vi "dscDIOOutputBit.vi"(6 "bit_val":enum8{"Lo", "Hi"}(ring), 8 "error in":errorcluster, 9 "bit":u8, 10 "port":u8, 11 "board":i16) -> (0 "error out":errorcluster, 3 "boardOut":i16)   [LabVIEW 2011, in "Diamond Universal Driver.lvlib"]
doc: "Sets the specified digital output bit of the specified port to the specified value (1 or 0) while leaving the other bits in their present states.\n\nSome boards (Diamond-MM, Diamond-MM-AT, Diamond-MM-16-AT, Opal-MM, Pearl-MM, Quartz-MM) do not have readback capability on the digital output ports. Therefore the driver maintains its own history of the last-written values to these ports, so that it can correctly modify only the bit of interest. In order for this function to work correctly, the driver must always know the present state of the digital output bits. This can only happen if you always use the driver for digital output operations. If you mix driver calls with direct I/O to the digital output ports, the bit operations can fail, since the driver will have no record of what your program has done directly."
uses:
  Diamond Universal Driver.lvlib
  Controls/error codes.ctl
  Instruments/WL OPC/Support/dlls/dscud.dll
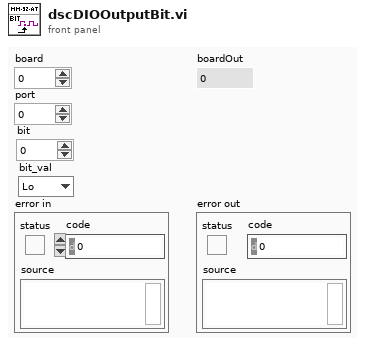
[diagram p1: front panel]
types:
  T1 = typedef "Diamond Universal Driver.lvlib/error codes.ctl" = enum8{"DE_NONE", "DE_HW_FAILURE", "DE_SW_FAILURE", "DE_HW_NOT_SUPPORTED", "DE_SW_NOT_SUPPORTED", "DE_INVALID_PARM", "DE_ALTERNATE_IN_PROGRESS", "DE_NONE_IN_PROGRESS", "DE_BUFFER_ROLLOVER", "DE_INVALID_ERROR_CODE", "DE_ALREADY_PAUSED", "DE_OVERFLOW", "DE_INVALID_FUNC", "DE_DSCUDH_INVALID", "DE_INVALID_BOARD", "DE_BOARD_LIMIT_REACHED", "DE_BOARD_BUSY", "DE_INVALID_WINDRVR_HANDLE", "DE_INVALID_WINDRVR_VERSION", "DE_BAD_WINDRVR_BOARD_INIT", "DE_OPERATION_TIMED_OUT", "DE_INVALID_WINDRVR_KP", "DE_THREAD_FAILURE"}
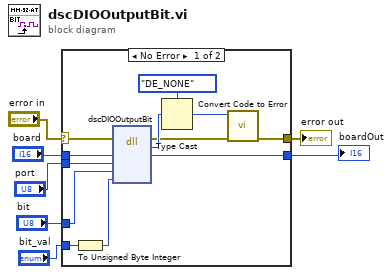
[diagram p0: block diagram]
diagram:
  n1 = case shown="No Error" "error in" {
    selector: "error in" -> [w16 w21]
    tunnel: "board" -> [w14 w20]
    tunnel: [w13 w20] -> w5
    tunnel: [w12 w21] -> w4
    tunnel: "port" -> [w11 _]
    tunnel: "bit" -> [w10 _]
    tunnel: "bit_val" -> [w9 _]
    frame No Error {
      n2 = To Unsigned Byte Integer(number=w9) -> (unsigned 8bit integer=w8:u8)
      n3 = dll-call lib="C:/Users/mrichardson/Documents/Web Based Version Control SW/Instruments/WL OPC/Support/dlls/dscud.dll" fn="dscDIOOutputBit"(error in=w16, "board"=w14, "port"=w11, "bit"=w10, "bit_val"=w8) -> (error out=w15:errorcluster, "error"=w17:u8, "board"=w13:i16)  [unwired: 5 in, 1 out]
      n4 = Type Cast(type=error_codes."DE_NONE" ("error codes"), x=w17) -> (*(type *) &x=w19:T1)
      n5 = call "Convert Code to Error.vi"("error in"=w15, "error codes"=w19) -> ("error out"=w12:errorcluster)  [unwired: 9 in]
    }
    frame Error {
    }
  }
  "boardOut" <- w5
  "error out" <- w4
